vi "Apply Filter_2D.vi"(9 "Column to Filter (0)":i32, 10 "Filter":string, 11 "Items to Filter":string[][](array[string])) -> (3 "Filtered Items":string[][](array[string]))   [LabVIEW 2015, in "E2E Tag Exchange editor node.lvclass"]
uses:
  E2E Tag Exchange editor node.lvclass
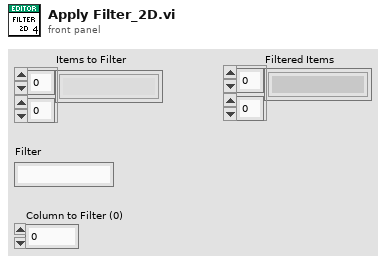
[diagram p1: front panel]
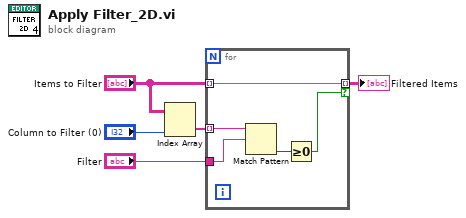
[diagram p0: block diagram]
diagram:
  n1 = Index Array(array="Items to Filter", index (col)="Column to Filter (0)") -> (element=w1:string[])  [unwired: 1 in]
  n2 = for {
    tunnel: "Items to Filter" -> [w9] mode=indexing
    tunnel: "Filter" -> [w10]
    tunnel: [w9] -> w4 mode=indexing if=w7
    tunnel: w1 -> [w6] mode=indexing
    n3 = Match Pattern(string=w6, regular expression=w10) -> (offset past match=w8:i32)  [unwired: 1 in, 3 out]
    n4 = Greater Or Equal To 0?(x=w8) -> (x >= 0?=w7:bool)
  }
  "Filtered Items" <- w4
